vi "test.vi"(7 "error in":errorcluster, 10 "RequestData":T1) -> (0 "error out":errorcluster, 2 "Parse Errors":string)   [LabVIEW 2023, in "MES.lvlib"]
uses:
  MES.lvlib
  <vilib>/xml/Load XML File.vi
  <vilib>/xml/Close Reference(Node).vi
  <vilib>/xml/Close Reference(NdList).vi
  <resource>/objmgr/DOMUserDefRef.rc
  <vilib>/xml/NI_XML.lvlib
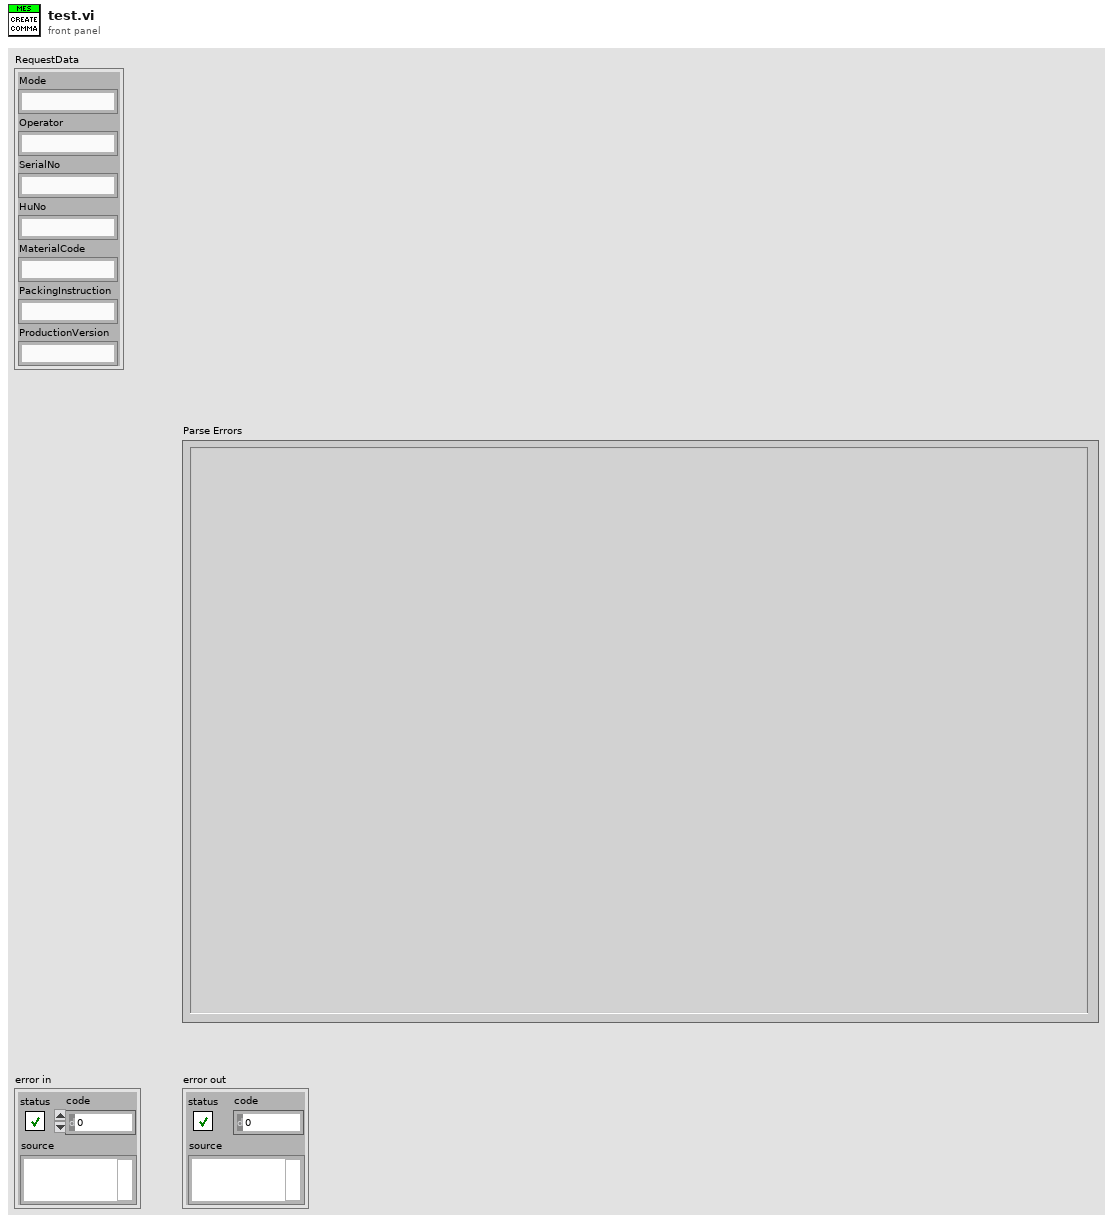
[diagram p1: front panel]
types:
  T1 = cluster{"Mode":string, "Operator":string, "SerialNo":string, "HuNo":string, "MaterialCode":string, "PackingInstruction":string, "ProductionVersion":string}
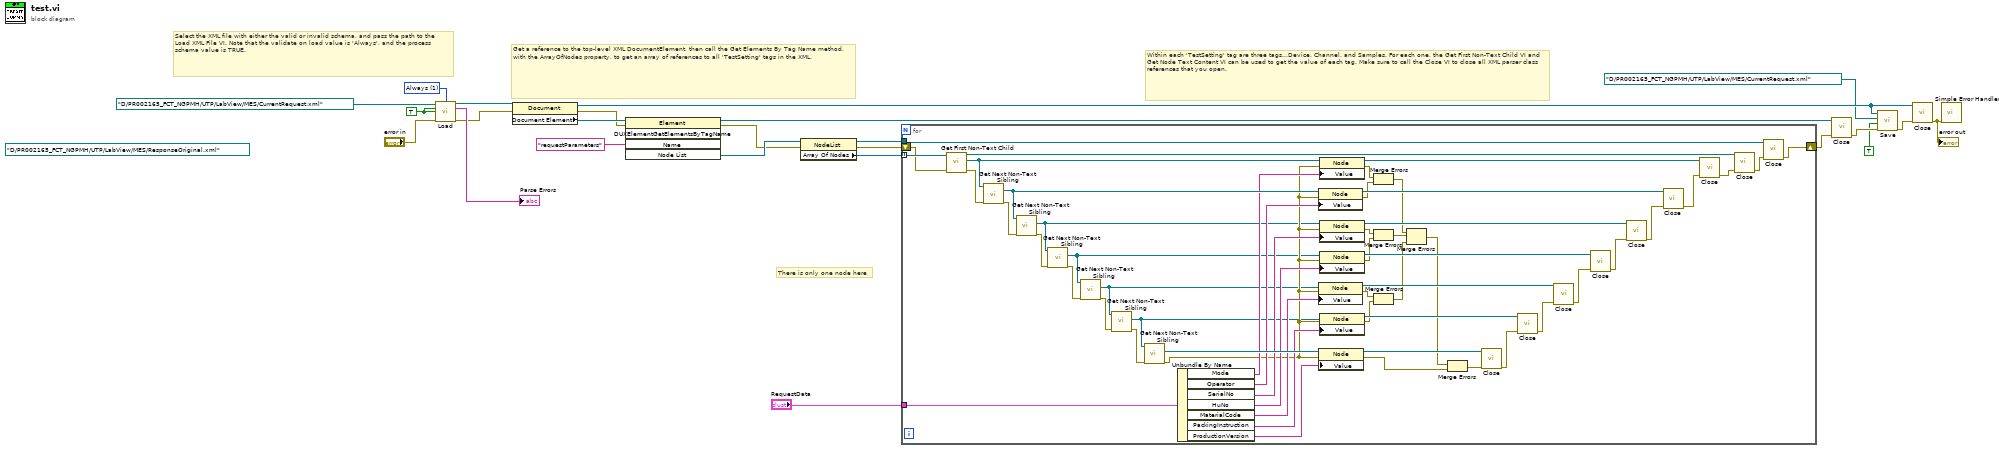
[diagram p0: block diagram]
diagram:
  (unwired) path "D:/PR002165_FCT_NGPMH/UTP/LabView/MES/ResponseOriginal.xml" ("file (use dialog)")
  w24 = 1 items=["Never", "Always", "Auto"] ("Validate On Load")
  w10 = TRUE ("Do Namespaces")
  # "There is only one node here"
  # "Within each 'TestSetting' tag are three tags...Device, Channel, and Samples. For each one, the Get First Non-Text Child VI and Get Node Text Content VI can be used to get the value of each tag. Make sure to call the Close VI to close all XML parser class references that you open."
  # "Get a reference to the top-level XML DocumentElement, then call the Get Elements By Tag Name method, with the ArrayOfNodes property, to get an array of references to all 'TestSetting' tags in the XML."
  # "Select the XML file with either the valid or invalid schema, and pass the path to the Load XML File VI. Note that the validate on load value is 'Always', and the process schema value is TRUE."
  n1 = call-poly <vilib>:"Load.vi"("path to XML document"=path "D:/PR002165_FCT_NGPMH/UTP/LabView/MES/CurrentRequest.xml" ("file (use dialog)"), "validate on load (Auto)"=w24, "process namespaces (False)"=w10, "process schema (False)"=w10, "error in (no error)"="error in") -> ("DOM document out"=w12:refnum<k20>, "parse errors"=→"Parse Errors":string, "error out"=w11:errorcluster)  [unwired: 2 in, 6 out]
  n2 = property class="Document"(reference=w12, error in=w11) -> (reference out=w5:refnum<k20>, error out=w20:errorcluster, "Document Element"=w21:refnum<k20>)
  n3 = invoke class="Element" method="DUXElementGetElementsByTagName"(reference=w21, error in=w20, "Name"="requestParameters" ("Node Name")) -> (reference out=w13:refnum<k20>, error out=w18:errorcluster, "Node List"=w19:refnum<k20>)  [unwired: 2 in, 2 out]
  n4 = property class="NodeList"(reference=w19, error in=w18) -> (reference out=w17:refnum<k20>, error out=w16:errorcluster, "Array Of Nodes"=w15:refnum<k20>[])
  n5 = for {
    tunnel: w15 -> [w73] mode=indexing
    tunnel: w17 -> [w75]
    shift-right: [w72] -> w14
    shift-left: w16 -> [w61]
    tunnel: "RequestData" -> [w29]
    n6 = call <vilib>:"Get First Non-Text Child.vi"("error in (no error)"=w61, "node in"=w73) -> ("error out"=w60:errorcluster, "child node"=w71:refnum<k20>, "node out"=w77:refnum<k20>)  [unwired: 7 out]
    n7 = call <vilib>:"Get Next Non-Text Sibling.vi"("error in (no error)"=w60, "node in"=w71) -> ("error out"=w59:errorcluster, "sibling node"=w69:refnum<k20>)  [unwired: 8 out]
    n8 = call <vilib>:"Get Next Non-Text Sibling.vi"("error in (no error)"=w59, "node in"=w69) -> ("error out"=w58:errorcluster, "sibling node"=w28:refnum<k20>)  [unwired: 8 out]
    n9 = call <vilib>:"Get Next Non-Text Sibling.vi"("error in (no error)"=w58, "node in"=w28) -> ("error out"=w57:errorcluster, "sibling node"=w27:refnum<k20>)  [unwired: 8 out]
    n10 = call <vilib>:"Get Next Non-Text Sibling.vi"("error in (no error)"=w57, "node in"=w27) -> ("error out"=w56:errorcluster, "sibling node"=w26:refnum<k20>)  [unwired: 8 out]
    n11 = call <vilib>:"Get Next Non-Text Sibling.vi"("error in (no error)"=w56, "node in"=w26) -> ("error out"=w55:errorcluster, "sibling node"=w25:refnum<k20>)  [unwired: 8 out]
    n12 = call <vilib>:"Get Next Non-Text Sibling.vi"("error in (no error)"=w55, "node in"=w25) -> ("error out"=w42:errorcluster, "sibling node"=w66:refnum<k20>)  [unwired: 8 out]
    n13 = Unbundle By Name(w29) -> ("Mode"=w49:string, "Operator"=w48:string, "SerialNo"=w47:string, "HuNo"=w46:string, "MaterialCode"=w45:string, "PackingInstruction"=w44:string, "ProductionVersion"=w43:string)
    n14 = property class="Node"(reference=w69, error in=w42, "Value"=w48) -> (reference out=w68:refnum<k20>, error out=w40:errorcluster)
    n15 = property class="Node"(reference=w26, error in=w42, "Value"=w45) -> (reference out=w63:refnum<k20>, error out=w37:errorcluster)
    n16 = property class="Node"(reference=w66, error in=w42, "Value"=w43) -> (reference out=w65:refnum<k20>, error out=w34:errorcluster)
    n17 = property class="Node"(reference=w71, error in=w42, "Value"=w49) -> (reference out=w70:refnum<k20>, error out=w41:errorcluster)
    n18 = property class="Node"(reference=w28, error in=w42, "Value"=w47) -> (reference out=w67:refnum<k20>, error out=w39:errorcluster)
    n19 = property class="Node"(reference=w27, error in=w42, "Value"=w46) -> (reference out=w62:refnum<k20>, error out=w38:errorcluster)
    n20 = property class="Node"(reference=w25, error in=w42, "Value"=w44) -> (reference out=w64:refnum<k20>, error out=w36:errorcluster)
    n21 = Merge Errors(w41, w40) -> (w32:errorcluster)
    n22 = Merge Errors(w39, w38) -> (w33:errorcluster)
    n23 = Merge Errors(w37, w36) -> (w31:errorcluster)
    n24 = Merge Errors(w32, w33, w31) -> (w30:errorcluster)
    n25 = Merge Errors(w30, w34) -> (w35:errorcluster)
    n26 = call-poly <vilib>:"Close.vi"("error in (no error)"=w35, "node"=w65) -> ("error out"=w54:errorcluster)  [unwired: 7 out]
    n27 = call-poly <vilib>:"Close.vi"("error in (no error)"=w54, "node"=w64) -> ("error out"=w53:errorcluster)  [unwired: 7 out]
    n28 = call-poly <vilib>:"Close.vi"("error in (no error)"=w53, "node"=w63) -> ("error out"=w52:errorcluster)  [unwired: 7 out]
    n29 = call-poly <vilib>:"Close.vi"("error in (no error)"=w52, "node"=w62) -> ("error out"=w51:errorcluster)  [unwired: 7 out]
    n30 = call-poly <vilib>:"Close.vi"("error in (no error)"=w51, "node"=w67) -> ("error out"=w50:errorcluster)  [unwired: 7 out]
    n31 = call-poly <vilib>:"Close.vi"("error in (no error)"=w50, "node"=w68) -> ("error out"=w78:errorcluster)  [unwired: 7 out]
    n32 = call-poly <vilib>:"Close.vi"("error in (no error)"=w78, "node"=w70) -> ("error out"=w76:errorcluster)  [unwired: 7 out]
    n33 = call-poly <vilib>:"Close.vi"("error in (no error)"=w76, "node"=w77) -> ("error out"=w74:errorcluster)  [unwired: 7 out]
    n34 = call-poly <vilib>:"Close.vi"("error in (no error)"=w74, "node list"=w75) -> ("error out"=w72:errorcluster)  [unwired: 7 out]
  }
  n35 = call-poly <vilib>:"Close.vi"("error in (no error)"=w14, "node"=w13) -> ("error out"=w4:errorcluster)  [unwired: 7 out]
  n36 = call <vilib>:"Save.vi"("error in (no error)"=w4, "overwrite file (True)"=TRUE, "XML file path"=path "D:/PR002165_FCT_NGPMH/UTP/LabView/MES/CurrentRequest.xml" ("file (use dialog)"), "DOM document in"=w5) -> ("error out"=w3:errorcluster)  [unwired: 5 in, 2 out]
  n37 = call-poly <vilib>:"Close.vi"("error in (no error)"=w3, "node"=w5) -> ("error out"=w7:errorcluster)  [unwired: 7 out]
  "error out" <- w7
  n38 = call <vilib>:"Simple Error Handler.vi"("error in (no error)"=w7) -> ()  [unwired: 4 in, 5 out]
